vi "getColor.vi"(0 "reference":refnum<class "Graphics.lvclass">, 5 "error in (no error)":errorcluster) -> (14 "reference out":refnum<class "Graphics.lvclass">, 15 "color":u32(colorbox), 19 "error out":errorcluster)   [LabVIEW 2012, in "Graphics.lvclass"]
doc: "Gets the current color"
uses:
  <resource>/Framework/Providers/Open_GDS/UML/Graphics_class/Graphics.lvclass
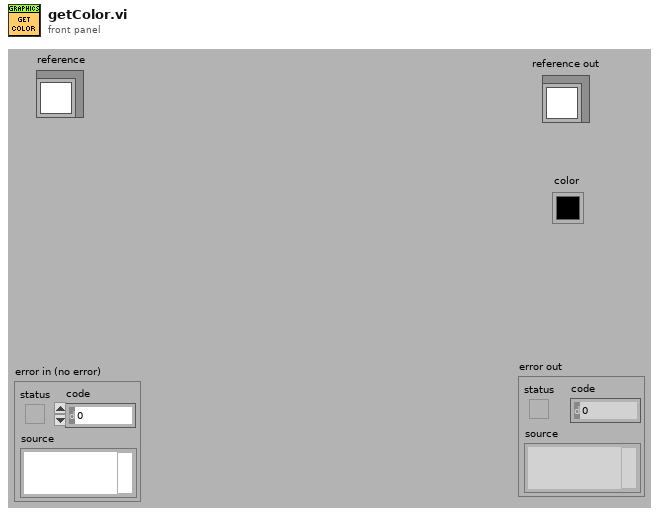
[diagram p1: front panel]
types:
  T1 = typedef "Graphics.lvclass/ObjectAttributes.ctl" = cluster{"drawColor":u32, "backgroundColor":u32, "font":T2, "fontType":T3, "picture":picture, "stroke":T4, "scaleX":dbl, "scaleY":dbl, "screenRef":refnum<vi>, "offsetX":dbl, "offsetY":dbl}
  T2 = typedef "Graphics.lvclass/FontType.ctl" = cluster{"Font Name:":string, "Size":i16, "Strikeout?":bool, "Italic?":bool, "Underline?":bool, "Outline?":bool, "Shadow?":bool, "Bold?":bool}
  T3 = typedef "Graphics.lvclass/LvFontType.ctl" = enum16{"User-specified Font", "Application Font", "System Font", "Dialog Font"}
  T4 = typedef "Graphics.lvclass/StrokeType.ctl" = enum16{"USE_DEFAULT", "SOLID", "DOTTED"}
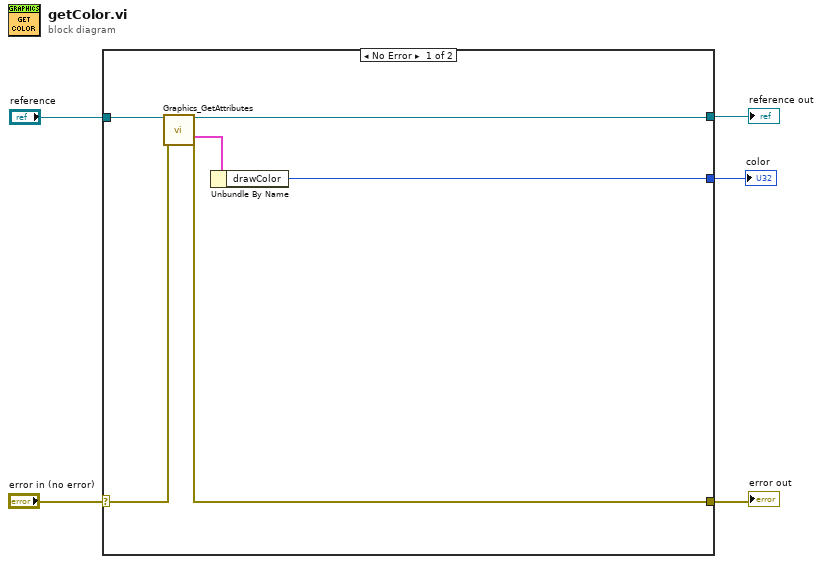
[diagram p0: block diagram]
diagram:
  n1 = case shown="No Error" "error in (no error)" {
    selector: "error in (no error)" -> [w11 w12]
    tunnel: "reference" -> [w10 w13]
    tunnel: [w8 w12] -> w3
    tunnel: [w9 w13] -> w2
    tunnel: [w7 _] -> w1
    frame No Error {
      n2 = call <resource>:"Graphics_GetAttributes.vi"("reference in"=w10, "error in (no error)"=w11) -> ("reference out"=w9:refnum<class "Graphics.lvclass">, "Data"=w6:T1, "error out"=w8:errorcluster)  [unwired: 1 in, 14 out]
      n3 = Unbundle By Name(w6) -> ("drawColor"=w7:u32)
    }
    frame Error {
    }
  }
  "reference out" <- w2
  "error out" <- w3
  "color" <- w1
